vi "Load Parameters.vi"(3 "error in":errorcluster, 5 "Subject Parameters File":path) -> (0 "error out":errorcluster, 1 "Subject Parameters":T1 {"Subject" items=["Subject 0", "Subject 1", "Subject 2", "Subject 3", "Subject 4", "Subject 5", "Subject 6", "Subject 7", "Subject 8", "Subject 9", "Subject 10", "Subject 11", "Subject 12", "Subject 13", "Subject 14", "Subject 15", "Subject 16", "Subject 17", "Subject 18", "Subject 19", "Subject 20", "Subject 21", "Subject 22", "Subject 23", "Subject 24", "Subject 25", "Subject 26", "Subject 27", "Subject 28", "Subject 29", "Subject 30", "Subject 31", "Subject 32", "Subject 33", "Subject 34", "Subject 35", "Subject 36", "Subject 37", "Subject 38", "Subject 39", "Subject 40"]}, 2 "Subject Parameters File":path)   [LabVIEW 2019]
uses:
  Controls/Subject Params.ctl
  Controls/Subject.ctl
  Controls/GPD Side Parameters.ctl
  Controls/Type Defs/Stim Parameters.ctl
  Controls/Stim off-half-ful.ctl
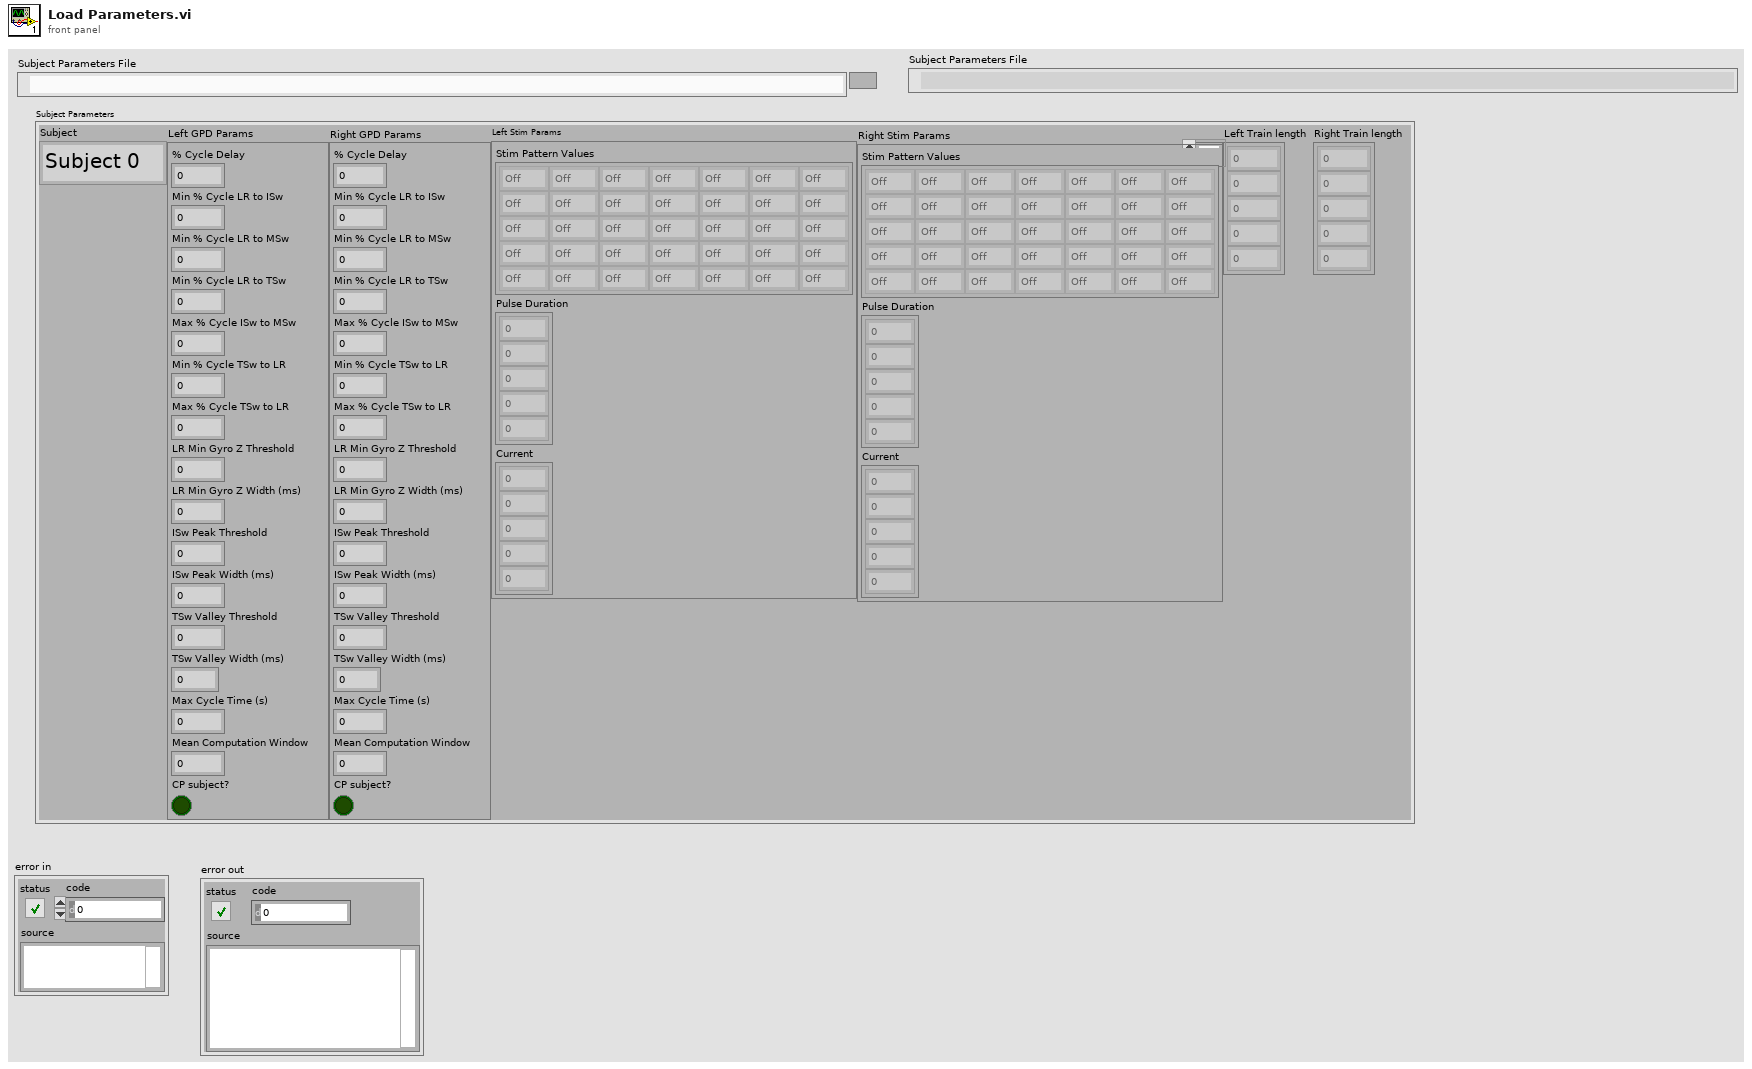
[diagram p1: front panel]
types:
  T1 = typedef "Subject Params.ctl" = cluster{"Subject":T2, "Left GPD Params":T3, "Right GPD Params":T3, "Left Stim Params":T4, "Right Stim Params":T4, "Left Train length":i64[], "Right Train length":i64[]}
  T2 = typedef "Subject.ctl" = u16
  T3 = typedef "GPD Side Parameters.ctl" = cluster{"% Cycle Delay":dbl, "Min % Cycle LR to ISw ":dbl, "Min % Cycle LR to MSw":dbl, "Min % Cycle LR to TSw":dbl, "Max % Cycle ISw to MSw":dbl, "Min % Cycle TSw to LR":dbl, "Max % Cycle TSw to LR":dbl, "LR Min Gyro Z Threshold":dbl, "LR Min Gyro Z Width":dbl, "ISw Peak Threshold":dbl, "ISw Peak Width":dbl, "TSw Valley Threshold":dbl, "TSw Valley Width (ms)":dbl, "Max Cycle Time (s)":dbl, "Mean Computation Window":dbl, "CP subject?":bool}
  T4 = typedef "Stim Parameters.ctl" = cluster{"Stim Pattern Values":T5[][], "Pulse Duration":i64[], "Current":i64[]}
  T5 = typedef "Stim off-half-ful.ctl" = enum16{"Off", "Half", "Full"}
  T6 = enum16{"open", "replace", "create", "open or create", "replace or create", "replace or create with confirmation"}
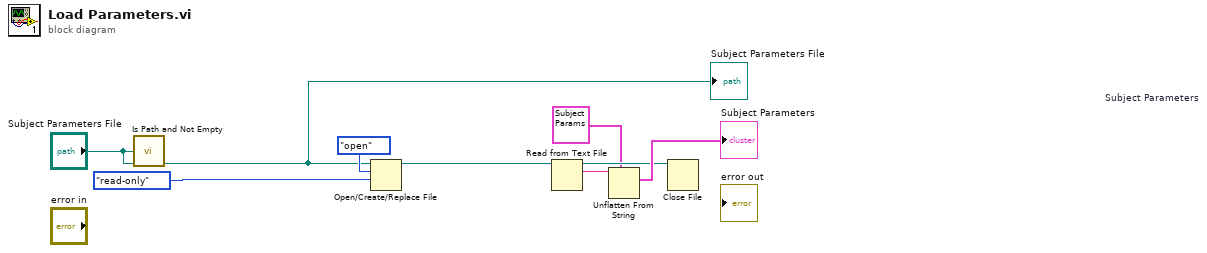
[diagram p0: block diagram]
diagram:
  w3 = T1 {"Subject"=0, "Left GPD Params"={"% Cycle Delay"=75.0, "Min % Cycle LR to ISw "=55.0, "Min % Cycle LR to MSw"=50.0, "Min % Cycle LR to TSw"=75.0, "Max % Cycle ISw to MSw"=10.0, "Min % Cycle TSw to LR"=2.5, "Max % Cycle TSw to LR"=75.0, "LR Min Gyro Z Threshold"=-0.3, "LR Min Gyro Z Width"=230.0, "ISw Peak Threshold"=0.6, "ISw Peak Width"=55.0, "TSw Valley Threshold"=-0.5, "TSw Valley Width (ms)"=55.0, "Max Cycle Time (s)"=1.3, "Mean Computation Window"=10.0, "CP subject?"=FALSE}, "Right GPD Params"={"% Cycle Delay"=75.0, "Min % Cycle LR to ISw "=55.0, "Min % Cycle LR to MSw"=50.0, "Min % Cycle LR to TSw"=75.0, "Max % Cycle ISw to MSw"=10.0, "Min % Cycle TSw to LR"=2.5, "Max % Cycle TSw to LR"=75.0, "LR Min Gyro Z Threshold"=-0.3, "LR Min Gyro Z Width"=230.0, "ISw Peak Threshold"=0.6, "ISw Peak Width"=55.0, "TSw Valley Threshold"=-0.5, "TSw Valley Width (ms)"=55.0, "Max Cycle Time (s)"=1.3, "Mean Computation Window"=10.0, "CP subject?"=FALSE}, "Left Stim Params"={"Stim Pattern Values"=[[enum."Full", enum."Half", enum."Off", enum."Off", enum."Off", enum."Off", enum."Half"], [enum."Full", enum."Off", enum."Off", enum."Off", enum."Off", enum."Half", enum."Half"], [enum."Half", enum."Full", enum."Off", enum."Full", enum."Off", enum."Off", enum."Full"], [enum."Half", enum."Off", enum."Off", enum."Half", enum."Full", enum."Full", enum."Full"], [enum."Off", enum."Full", enum."Half", enum."Half", enum."Off", enum."Off", enum."Off"]], "Pulse Duration"=[20, 200, 200, 200, 200], "Current"=[20, 20, 20, 20, 20]}, "Right Stim Params"={"Stim Pattern Values"=[[enum."Full", enum."Half", enum."Off", enum."Off", enum."Off", enum."Off", enum."Half"], [enum."Full", enum."Off", enum."Off", enum."Off", enum."Off", enum."Half", enum."Half"], [enum."Half", enum."Full", enum."Off", enum."Full", enum."Off", enum."Off", enum."Full"], [enum."Half", enum."Off", enum."Off", enum."Half", enum."Full", enum."Full", enum."Full"], [enum."Off", enum."Full", enum."Half", enum."Half", enum."Off", enum."Off", enum."Off"]], "Pulse Duration"=[200, 200, 200, 200, 200], "Current"=[200, 200, 200, 200, 200]}, "Left Train length"=[300, 300, 300, 300, 300], "Right Train length"=[300, 300, 300, 300, 300]}  # Subject Parameters
  n1 = call <vilib>:"Is Path and Not Empty.vi"("path"="Subject Parameters File") -> ()  [unwired: 4 in, 1 out]
  n2 = Open/Create/Replace File(file path (use dialog)="Subject Parameters File", operation (0:open)=T6."open", access (0:read/write)=enum16{"read/write", "read-only", "write-only"}."read-only") -> (refnum out=w4:refnum<file>)  [unwired: 3 in, 2 out]
  n3 = Read from Text File(file (use dialog)=w4) -> (refnum out=w6:refnum<file>, text=w8:string)  [unwired: 3 in, 2 out]
  n4 = Unflatten From String(type=w3, binary string=w8) -> (value=→"Subject Parameters":T1)  [unwired: 3 in, 2 out]
  n5 = Close File(refnum=w6) -> ()  [unwired: 1 in, 2 out]
  "Subject Parameters File" <- "Subject Parameters File"
